vi "test.vi"() -> ()   [LabVIEW 2009]
uses:
  <vilib>/Utility/file.llb/Read From Spreadsheet File (DBL).vi
  <vilib>/Utility/file.llb/Write To Spreadsheet File (DBL).vi
panel:
  out "XY Graph 3":cluster{dbl[], dbl[]}(graph)
  in  "Open Path":path
  in  "Save Path":path
  out "XY Graph":cluster{dbl[], dbl[]}(graph)
  out "XY Graph 2":cluster{dbl[], dbl[]}(graph)
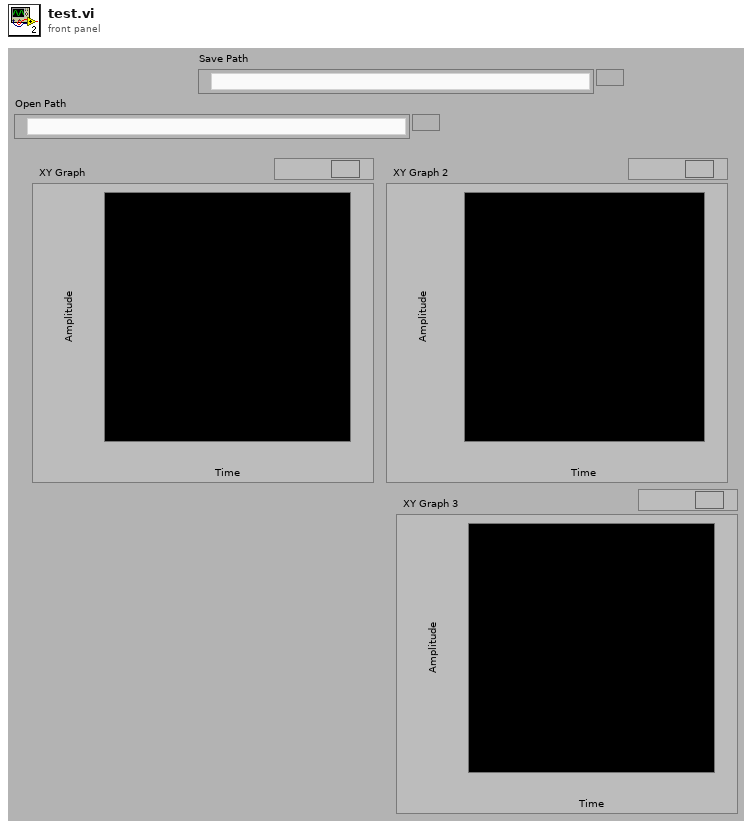
[diagram p1: front panel]
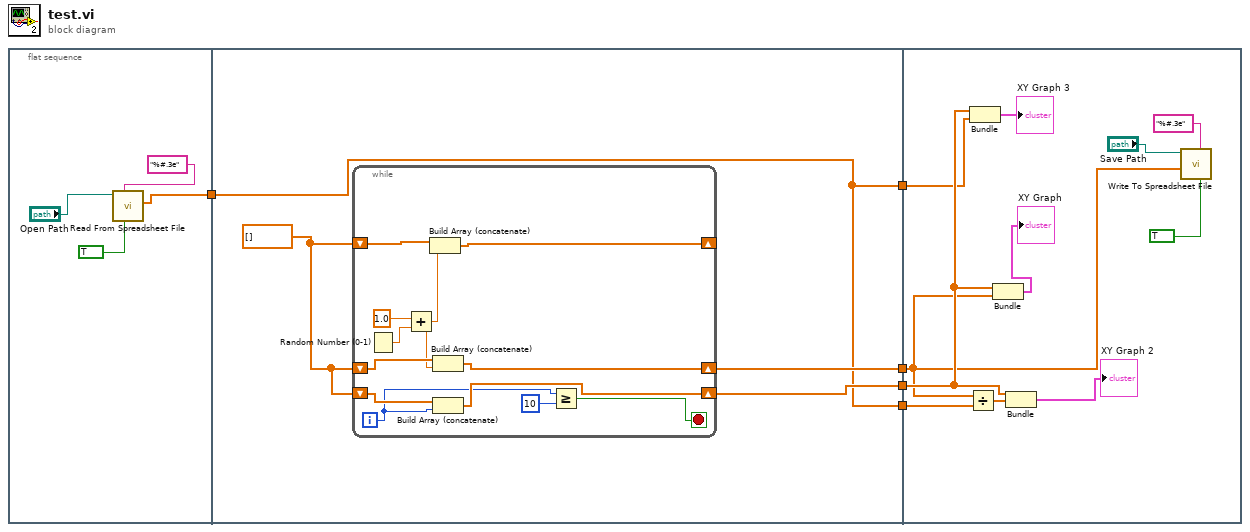
[diagram p0: block diagram]
diagram:
  n1 = flat-sequence {
    tunnel: [w6] -> w3
    tunnel: [w12] -> w5
    tunnel: [w11] -> w4
    tunnel: w3 -> [w10]
    tunnel: [w10] -> w2
    tunnel: [w10] -> w1
    tunnel: w5 -> [w29]
    tunnel: w4 -> [w26]
    tunnel: w2 -> [w28]
    tunnel: w1 -> [w27]
    frame #0 {
      n2 = call-poly <vilib>:"Read From Spreadsheet File.vi"("transpose (no:F)"=TRUE, "format (%.3f)"="%#.3e", "file path (dialog if empty)"="Open Path") -> ("first row"=w6:dbl[])  [unwired: 4 in, 4 out]
    }
    frame #1 {
      w13 = dbl[] []
      n3 = while {
        shift-right: [w24] -> _
        shift-left: w13 -> [w25]
        shift-right: [w22] -> w11
        shift-left: w13 -> [w23]
        shift-right: [w18] -> w12
        shift-left: w13 -> [w19]
        i -> [w16]
        stop <- w20 stop-if-true
        n4 = Random Number (0-1)() -> (number: 0 to 1=w14:dbl)
        n5 = Add(x=1.0 ("y"), y=w14) -> (x+y=w15:dbl)
        n6 = Build Array (concatenate)(w25, w15) -> (w24:dbl[])
        n7 = Build Array (concatenate)(w23, w15) -> (w22:dbl[])
        n8 = Build Array (concatenate)(w19, w16) -> (w18:dbl[])
        n9 = Greater Or Equal?(x=w16, y=10) -> (x >= y?=w20:bool)
      }
    }
    frame #2 {
      n10 = Divide(x=w26, y=w28) -> (x/y=w33:dbl[])
      n11 = Bundle(w29, "first row"=w27) -> (→"XY Graph 3":cluster{dbl[], "first row":dbl[]})  [unwired: 1 in]
      n12 = Bundle(w29, w26) -> (→"XY Graph":cluster{dbl[], dbl[]})  [unwired: 1 in]
      n13 = Bundle(w29, w33) -> (→"XY Graph 2":cluster{dbl[], dbl[]})  [unwired: 1 in]
      n14 = call-poly <vilib>:"Write To Spreadsheet File.vi"("transpose? (no:F)"=TRUE, "format (%.3f)"="%#.3e", "1D data"=w26, "file path (dialog if empty)"="Save Path") -> ()  [unwired: 4 in, 1 out]
    }
  }
